vi "S7COMM - Setup Communication.vi"(8 "error in (no error)":errorcluster, 11 "S7NetCom in":refnum<class "S7NetCom.lvclass">) -> (0 "error out":errorcluster, 2 "S7 PDU":u8[](array[numeric]) format="%02x", 3 "S7NetCom out":refnum<class "S7NetCom.lvclass">)   [LabVIEW 2014, in "S7NetCom.lvclass"]
doc: "____\nCopyright (c) 2019 Hampel Software Engineering (HSE), released under BSD license. More info can be found on https://dokuwiki.hampel-soft.com/code/hse/s7netcom. Original code published by Marc Christenson, Sisu Devices."
uses:
  S7NetCom.lvclass
  Controls/S7NetCom_HexByteArray.ctl
  Controls/S7NetCom_HexByte.ctl
  S7NetCom.lvclass/S7NetCom.ctl
  TPKT/TPKT - Write Packet.vi
  COTP/COTP - Add Header.vi
  COTP/COTP - Validate Response Header.vi
  S7COMM - Create JOB Message Header.vi
  TPKT/TPKT - Add Header.vi
  Accessors/Get Timeout.vi
  Accessors/Get TCP Ref.vi
  Accessors/Set TCP Ref.vi
  COTP/COTP - Header for Data Transfer--constant.vi
  COTP/COTP - Response Header Mismatch--error.vi
  S7COMM - Header - Protocol ID--constant.vi
  TPKT/TPKT - Header Bytes 1 and 2--constant.vi
  TPKT/TPKT - Read Packet.vi
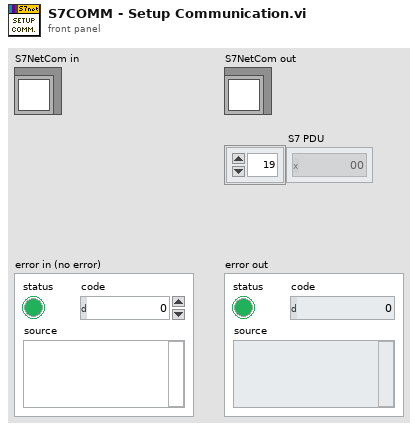
[diagram p1: front panel]
types:
  T1 = typedef "S7NetCom.lvclass/S7NetCom_HexByteArray.ctl" = T2[]
  T2 = typedef "S7NetCom.lvclass/S7NetCom_HexByte.ctl" = u8
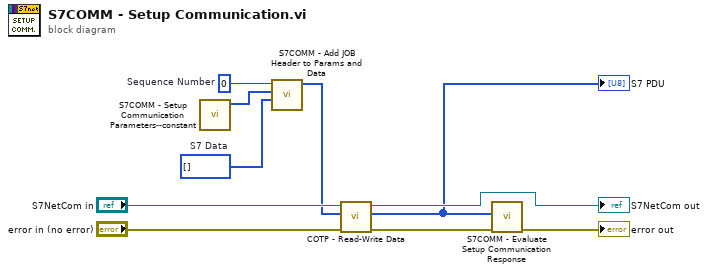
[diagram p0: block diagram]
diagram:
  w5 = T1 []  # S7 Data
  w6 = u16 0  # Sequence Number
  n1 = call "S7COMM - Setup Communication Parameters--constant.vi"() -> ("S7PDU \"Setup Communication\" Parameters"=w8:T1)  [unwired: 11 in]
  n2 = call "S7COMM - Add JOB Header to Params and Data.vi"("S7 Data"=w5, "S7 Parameters"=w8, "Sequence Number"=w6) -> ("S7 PDU"=w7:T1)  [unwired: 8 in]
  n3 = call "COTP - Read-Write Data.vi"("error in (no error)"="error in (no error)", "S7 PDU in"=w7, "S7 in"="S7NetCom in") -> ("error out"=w4:errorcluster, "S7 PDU out"=w1:T1, "S7 out"=→"S7NetCom out":refnum<class "S7NetCom.lvclass">)  [unwired: 6 in]
  "S7 PDU" <- w1
  n4 = call "S7COMM - Evaluate Setup Communication Response.vi"("error in (no error)"=w4, "S7 PDU"=w1) -> ("error out"=→"error out":errorcluster)  [unwired: 9 in]
